vi "DDS_Clock.vi"() -> ()   [LabVIEW 2016] (continued)
"f1 [Hz] CH0"=312200000.0}, {"total time[ms]"=23.050000000000193, "f1 [Hz] CH0"=312200000.0}, {"total time[ms]"=23.100000000000193, "f1 [Hz] CH0"=312400000.0}, {"total time[ms]"=23.100000000000193, "f1 [Hz] CH0"=312400000.0}, {"total time[ms]"=23.150000000000194, "f1 [Hz] CH0"=312600000.0}, {"total time[ms]"=23.150000000000194, "f1 [Hz] CH0"=312600000.0}, {"total time[ms]"=23.200000000000195, "f1 [Hz] CH0"=312800000.0}, {"total time[ms]"=23.200000000000195, "f1 [Hz] CH0"=312800000.0}, {"total time[ms]"=23.250000000000195, "f1 [Hz] CH0"=313000000.0}, {"total time[ms]"=23.250000000000195, "f1 [Hz] CH0"=313000000.0}, {"total time[ms]"=23.300000000000196, "f1 [Hz] CH0"=313200000.0}, {"total time[ms]"=23.300000000000196, "f1 [Hz] CH0"=313200000.0}, {"total time[ms]"=23.350000000000197, "f1 [Hz] CH0"=313400000.0}, {"total time[ms]"=23.350000000000197, "f1 [Hz] CH0"=313400000.0}, {"total time[ms]"=23.400000000000198, "f1 [Hz] CH0"=313600000.0}, {"total time[ms]"=23.400000000000198, "f1 [Hz] CH0"=313600000.0}, {"total time[ms]"=23.4500000000002, "f1 [Hz] CH0"=313800000.0}, {"total time[ms]"=23.4500000000002, "f1 [Hz] CH0"=313800000.0}, {"total time[ms]"=23.5000000000002, "f1 [Hz] CH0"=314000000.0}, {"total time[ms]"=23.5000000000002, "f1 [Hz] CH0"=314000000.0}, {"total time[ms]"=23.5500000000002, "f1 [Hz] CH0"=314200000.0}, {"total time[ms]"=23.5500000000002, "f1 [Hz] CH0"=314200000.0}, {"total time[ms]"=23.6000000000002, "f1 [Hz] CH0"=314400000.0}, {"total time[ms]"=23.6000000000002, "f1 [Hz] CH0"=314400000.0}, {"total time[ms]"=23.6500000000002, "f1 [Hz] CH0"=314600000.0}, {"total time[ms]"=23.6500000000002, "f1 [Hz] CH0"=314600000.0}, {"total time[ms]"=23.700000000000202, "f1 [Hz] CH0"=314800000.0}, {"total time[ms]"=23.700000000000202, "f1 [Hz] CH0"=314800000.0}, {"total time[ms]"=23.750000000000203, "f1 [Hz] CH0"=315000000.0}, {"total time[ms]"=23.750000000000203, "f1 [Hz] CH0"=315000000.0}, {"total time[ms]"=23.800000000000203, "f1 [Hz] CH0"=315200000.0}, {"total time[ms]"=23.800000000000203, "f1 [Hz] CH0"=315200000.0}, {"total time[ms]"=23.850000000000204, "f1 [Hz] CH0"=315400000.0}, {"total time[ms]"=23.850000000000204, "f1 [Hz] CH0"=315400000.0}, {"total time[ms]"=23.900000000000205, "f1 [Hz] CH0"=315600000.0}, {"total time[ms]"=23.900000000000205, "f1 [Hz] CH0"=315600000.0}, {"total time[ms]"=23.950000000000205, "f1 [Hz] CH0"=315800000.0}, {"total time[ms]"=23.950000000000205, "f1 [Hz] CH0"=315800000.0}, {"total time[ms]"=24.000000000000206, "f1 [Hz] CH0"=316000000.0}, {"total time[ms]"=24.000000000000206, "f1 [Hz] CH0"=316000000.0}, {"total time[ms]"=24.050000000000207, "f1 [Hz] CH0"=316200000.0}, {"total time[ms]"=24.050000000000207, "f1 [Hz] CH0"=316200000.0}, {"total time[ms]"=24.100000000000207, "f1 [Hz] CH0"=316400000.0}, {"total time[ms]"=24.100000000000207, "f1 [Hz] CH0"=316400000.0}, {"total time[ms]"=24.150000000000208, "f1 [Hz] CH0"=316600000.0}, {"total time[ms]"=24.150000000000208, "f1 [Hz] CH0"=316600000.0}, {"total time[ms]"=24.20000000000021, "f1 [Hz] CH0"=316800000.0}, {"total time[ms]"=24.20000000000021, "f1 [Hz] CH0"=316800000.0}, {"total time[ms]"=24.25000000000021, "f1 [Hz] CH0"=317000000.0}, {"total time[ms]"=24.25000000000021, "f1 [Hz] CH0"=317000000.0}, {"total time[ms]"=24.30000000000021, "f1 [Hz] CH0"=317200000.0}, {"total time[ms]"=24.30000000000021, "f1 [Hz] CH0"=317200000.0}, {"total time[ms]"=24.35000000000021, "f1 [Hz] CH0"=317400000.0}, {"total time[ms]"=24.35000000000021, "f1 [Hz] CH0"=317400000.0}, {"total time[ms]"=24.40000000000021, "f1 [Hz] CH0"=317600000.0}, {"total time[ms]"=24.40000000000021, "f1 [Hz] CH0"=317600000.0}, {"total time[ms]"=24.450000000000212, "f1 [Hz] CH0"=317800000.0}, {"total time[ms]"=24.450000000000212, "f1 [Hz] CH0"=317800000.0}, {"total time[ms]"=24.500000000000213, "f1 [Hz] CH0"=318000000.0}, {"total time[ms]"=24.500000000000213, "f1 [Hz] CH0"=318000000.0}, {"total time[ms]"=24.550000000000214, "f1 [Hz] CH0"=318200000.0}, {"total time[ms]"=24.550000000000214, "f1 [Hz] CH0"=318200000.0}, {"total time[ms]"=24.600000000000215, "f1 [Hz] CH0"=318400000.0}, {"total time[ms]"=24.600000000000215, "f1 [Hz] CH0"=318400000.0}, {"total time[ms]"=24.650000000000215, "f1 [Hz] CH0"=318600000.0}, {"total time[ms]"=24.650000000000215, "f1 [Hz] CH0"=318600000.0}, {"total time[ms]"=24.700000000000216, "f1 [Hz] CH0"=318800000.0}, {"total time[ms]"=24.700000000000216, "f1 [Hz] CH0"=318800000.0}, {"total time[ms]"=24.750000000000217, "f1 [Hz] CH0"=319000000.0}, {"total time[ms]"=24.750000000000217, "f1 [Hz] CH0"=319000000.0}, {"total time[ms]"=24.800000000000217, "f1 [Hz] CH0"=319200000.0}, {"total time[ms]"=24.800000000000217, "f1 [Hz] CH0"=319200000.0}, {"total time[ms]"=24.850000000000218, "f1 [Hz] CH0"=319400000.0}, {"total time[ms]"=24.850000000000218, "f1 [Hz] CH0"=319400000.0}, {"total time[ms]"=24.90000000000022, "f1 [Hz] CH0"=319600000.0}, {"total time[ms]"=24.90000000000022, "f1 [Hz] CH0"=319600000.0}, {"total time[ms]"=24.95000000000022, "f1 [Hz] CH0"=319800000.0}, {"total time[ms]"=24.95000000000022, "f1 [Hz] CH0"=319800000.0}, {"total time[ms]"=25.00000000000022, "f1 [Hz] CH0"=320000000.0}, {"total time[ms]"=25.00000000000022, "f1 [Hz] CH0"=320000000.0}, {"total time[ms]"=25.05000000000022, "f1 [Hz] CH0"=319800000.0}, {"total time[ms]"=25.05000000000022, "f1 [Hz] CH0"=319800000.0}, {"total time[ms]"=25.10000000000022, "f1 [Hz] CH0"=319600000.0}, {"total time[ms]"=25.10000000000022, "f1 [Hz] CH0"=319600000.0}, {"total time[ms]"=25.150000000000222, "f1 [Hz] CH0"=319400000.0}, {"total time[ms]"=25.150000000000222, "f1 [Hz] CH0"=319400000.0}, {"total time[ms]"=25.200000000000223, "f1 [Hz] CH0"=319200000.0}, {"total time[ms]"=25.200000000000223, "f1 [Hz] CH0"=319200000.0}, {"total time[ms]"=25.250000000000224, "f1 [Hz] CH0"=319000000.0}, {"total time[ms]"=25.250000000000224, "f1 [Hz] CH0"=319000000.0}, {"total time[ms]"=25.300000000000225, "f1 [Hz] CH0"=318800000.0}, {"total time[ms]"=25.300000000000225, "f1 [Hz] CH0"=318800000.0}, {"total time[ms]"=25.350000000000225, "f1 [Hz] CH0"=318600000.0}, {"total time[ms]"=25.350000000000225, "f1 [Hz] CH0"=318600000.0}, {"total time[ms]"=25.400000000000226, "f1 [Hz] CH0"=318400000.0}, {"total time[ms]"=25.400000000000226, "f1 [Hz] CH0"=318400000.0}, {"total time[ms]"=25.450000000000227, "f1 [Hz] CH0"=318200000.0}, {"total time[ms]"=25.450000000000227, "f1 [Hz] CH0"=318200000.0}, {"total time[ms]"=25.500000000000227, "f1 [Hz] CH0"=318000000.0}, {"total time[ms]"=25.500000000000227, "f1 [Hz] CH0"=318000000.0}, {"total time[ms]"=25.550000000000228, "f1 [Hz] CH0"=317800000.0}, {"total time[ms]"=25.550000000000228, "f1 [Hz] CH0"=317800000.0}, {"total time[ms]"=25.60000000000023, "f1 [Hz] CH0"=317600000.0}, {"total time[ms]"=25.60000000000023, "f1 [Hz] CH0"=317600000.0}, {"total time[ms]"=25.65000000000023, "f1 [Hz] CH0"=317400000.0}, {"total time[ms]"=25.65000000000023, "f1 [Hz] CH0"=317400000.0}, {"total time[ms]"=25.70000000000023, "f1 [Hz] CH0"=317200000.0}, {"total time[ms]"=25.70000000000023, "f1 [Hz] CH0"=317200000.0}, {"total time[ms]"=25.75000000000023, "f1 [Hz] CH0"=317000000.0}, {"total time[ms]"=25.75000000000023, "f1 [Hz] CH0"=317000000.0}, {"total time[ms]"=25.80000000000023, "f1 [Hz] CH0"=316800000.0}, {"total time[ms]"=25.80000000000023, "f1 [Hz] CH0"=316800000.0}, {"total time[ms]"=25.850000000000232, "f1 [Hz] CH0"=316600000.0}, {"total time[ms]"=25.850000000000232, "f1 [Hz] CH0"=316600000.0}, {"total time[ms]"=25.900000000000233, "f1 [Hz] CH0"=316400000.0}, {"total time[ms]"=25.900000000000233, "f1 [Hz] CH0"=316400000.0}, {"total time[ms]"=25.950000000000234, "f1 [Hz] CH0"=316200000.0}, {"total time[ms]"=25.950000000000234, "f1 [Hz] CH0"=316200000.0}, {"total time[ms]"=26.000000000000234, "f1 [Hz] CH0"=316000000.0}, {"total time[ms]"=26.000000000000234, "f1 [Hz] CH0"=316000000.0}, {"total time[ms]"=26.050000000000235, "f1 [Hz] CH0"=315800000.0}, {"total time[ms]"=26.050000000000235, "f1 [Hz] CH0"=315800000.0}, {"total time[ms]"=26.100000000000236, "f1 [Hz] CH0"=315600000.0}, {"total time[ms]"=26.100000000000236, "f1 [Hz] CH0"=315600000.0}, {"total time[ms]"=26.150000000000237, "f1 [Hz] CH0"=315400000.0}, {"total time[ms]"=26.150000000000237, "f1 [Hz] CH0"=315400000.0}, {"total time[ms]"=26.200000000000237, "f1 [Hz] CH0"=315200000.0}, {"total time[ms]"=26.200000000000237, "f1 [Hz] CH0"=315200000.0}, {"total time[ms]"=26.250000000000238, "f1 [Hz] CH0"=315000000.0}, {"total time[ms]"=26.250000000000238, "f1 [Hz] CH0"=315000000.0}, {"total time[ms]"=26.30000000000024, "f1 [Hz] CH0"=314800000.0}, {"total time[ms]"=26.30000000000024, "f1 [Hz] CH0"=314800000.0}, {"total time[ms]"=26.35000000000024, "f1 [Hz] CH0"=314600000.0}, {"total time[ms]"=26.35000000000024, "f1 [Hz] CH0"=314600000.0}, {"total time[ms]"=26.40000000000024, "f1 [Hz] CH0"=314400000.0}, {"total time[ms]"=26.40000000000024, "f1 [Hz] CH0"=314400000.0}, {"total time[ms]"=26.45000000000024, "f1 [Hz] CH0"=314200000.0}, {"total time[ms]"=26.45000000000024, "f1 [Hz] CH0"=314200000.0}, {"total time[ms]"=26.50000000000024, "f1 [Hz] CH0"=314000000.0}, {"total time[ms]"=26.50000000000024, "f1 [Hz] CH0"=314000000.0}, {"total time[ms]"=26.550000000000242, "f1 [Hz] CH0"=313800000.0}, {"total time[ms]"=26.550000000000242, "f1 [Hz] CH0"=313800000.0}, {"total time[ms]"=26.600000000000243, "f1 [Hz] CH0"=313600000.0}, {"total time[ms]"=26.600000000000243, "f1 [Hz] CH0"=313600000.0}, {"total time[ms]"=26.650000000000244, "f1 [Hz] CH0"=313400000.0}, {"total time[ms]"=26.650000000000244, "f1 [Hz] CH0"=313400000.0}, {"total time[ms]"=26.700000000000244, "f1 [Hz] CH0"=313200000.0}, {"total time[ms]"=26.700000000000244, "f1 [Hz] CH0"=313200000.0}, {"total time[ms]"=26.750000000000245, "f1 [Hz] CH0"=313000000.0}, {"total time[ms]"=26.750000000000245, "f1 [Hz] CH0"=313000000.0}, {"total time[ms]"=26.800000000000246, "f1 [Hz] CH0"=312800000.0}, {"total time[ms]"=26.800000000000246, "f1 [Hz] CH0"=312800000.0}, {"total time[ms]"=26.850000000000247, "f1 [Hz] CH0"=312600000.0}, {"total time[ms]"=26.850000000000247, "f1 [Hz] CH0"=312600000.0}, {"total time[ms]"=26.900000000000247, "f1 [Hz] CH0"=312400000.0}, {"total time[ms]"=26.900000000000247, "f1 [Hz] CH0"=312400000.0}, {"total time[ms]"=26.950000000000248, "f1 [Hz] CH0"=312200000.0}, {"total time[ms]"=26.950000000000248, "f1 [Hz] CH0"=312200000.0}, {"total time[ms]"=27.00000000000025, "f1 [Hz] CH0"=312000000.0}, {"total time[ms]"=27.00000000000025, "f1 [Hz] CH0"=312000000.0}, {"total time[ms]"=27.05000000000025, "f1 [Hz] CH0"=311800000.0}, {"total time[ms]"=27.05000000000025, "f1 [Hz] CH0"=311800000.0}, {"total time[ms]"=27.10000000000025, "f1 [Hz] CH0"=311600000.0}, {"total time[ms]"=27.10000000000025, "f1 [Hz] CH0"=311600000.0}, {"total time[ms]"=27.15000000000025, "f1 [Hz] CH0"=311400000.0}, {"total time[ms]"=27.15000000000025, "f1 [Hz] CH0"=311400000.0}, {"total time[ms]"=27.20000000000025, "f1 [Hz] CH0"=311200000.0}, {"total time[ms]"=27.20000000000025, "f1 [Hz] CH0"=311200000.0}, {"total time[ms]"=27.250000000000252, "f1 [Hz] CH0"=311000000.0}, {"total time[ms]"=27.250000000000252, "f1 [Hz] CH0"=311000000.0}, {"total time[ms]"=27.300000000000253, "f1 [Hz] CH0"=310800000.0}, {"total time[ms]"=27.300000000000253, "f1 [Hz] CH0"=310800000.0}, {"total time[ms]"=27.350000000000254, "f1 [Hz] CH0"=310600000.0}, {"total time[ms]"=27.350000000000254, "f1 [Hz] CH0"=310600000.0}, {"total time[ms]"=27.400000000000254, "f1 [Hz] CH0"=310400000.0}, {"total time[ms]"=27.400000000000254, "f1 [Hz] CH0"=310400000.0}, {"total time[ms]"=27.450000000000255, "f1 [Hz] CH0"=310200000.0}, {"total time[ms]"=27.450000000000255, "f1 [Hz] CH0"=310200000.0}, {"total time[ms]"=27.500000000000256, "f1 [Hz] CH0"=310000000.0}, {"total time[ms]"=27.500000000000256, "f1 [Hz] CH0"=310000000.0}, {"total time[ms]"=27.550000000000257, "f1 [Hz] CH0"=309800000.0}, {"total time[ms]"=27.550000000000257, "f1 [Hz] CH0"=309800000.0}, {"total time[ms]"=27.600000000000257, "f1 [Hz] CH0"=309600000.0}, {"total time[ms]"=27.600000000000257, "f1 [Hz] CH0"=309600000.0}, {"total time[ms]"=27.650000000000258, "f1 [Hz] CH0"=309400000.0}, {"total time[ms]"=27.650000000000258, "f1 [Hz] CH0"=309400000.0}, {"total time[ms]"=27.70000000000026, "f1 [Hz] CH0"=309200000.0}, {"total time[ms]"=27.70000000000026, "f1 [Hz] CH0"=309200000.0}, {"total time[ms]"=27.75000000000026, "f1 [Hz] CH0"=309000000.0}, {"total time[ms]"=27.75000000000026, "f1 [Hz] CH0"=309000000.0}, {"total time[ms]"=27.80000000000026, "f1 [Hz] CH0"=308800000.0}, {"total time[ms]"=27.80000000000026, "f1 [Hz] CH0"=308800000.0}, {"total time[ms]"=27.85000000000026, "f1 [Hz] CH0"=308600000.0}, {"total time[ms]"=27.85000000000026, "f1 [Hz] CH0"=308600000.0}, {"total time[ms]"=27.90000000000026, "f1 [Hz] CH0"=308400000.0}, {"total time[ms]"=27.90000000000026, "f1 [Hz] CH0"=308400000.0}, {"total time[ms]"=27.950000000000262, "f1 [Hz] CH0"=308200000.0}, {"total time[ms]"=27.950000000000262, "f1 [Hz] CH0"=308200000.0}, {"total time[ms]"=28.000000000000263, "f1 [Hz] CH0"=308000000.0}, {"total time[ms]"=28.000000000000263, "f1 [Hz] CH0"=308000000.0}, {"total time[ms]"=28.050000000000264, "f1 [Hz] CH0"=307800000.0}, {"total time[ms]"=28.050000000000264, "f1 [Hz] CH0"=307800000.0}, {"total time[ms]"=28.100000000000264, "f1 [Hz] CH0"=307600000.0}, {"total time[ms]"=28.100000000000264, "f1 [Hz] CH0"=307600000.0}, {"total time[ms]"=28.150000000000265, "f1 [Hz] CH0"=307400000.0}, {"total time[ms]"=28.150000000000265, "f1 [Hz] CH0"=307400000.0}, {"total time[ms]"=28.200000000000266, "f1 [Hz] CH0"=307200000.0}, {"total time[ms]"=28.200000000000266, "f1 [Hz] CH0"=307200000.0}, {"total time[ms]"=28.250000000000266, "f1 [Hz] CH0"=307000000.0}, {"total time[ms]"=28.250000000000266, "f1 [Hz] CH0"=307000000.0}, {"total time[ms]"=28.300000000000267, "f1 [Hz] CH0"=306800000.0}, {"total time[ms]"=28.300000000000267, "f1 [Hz] CH0"=306800000.0}, {"total time[ms]"=28.350000000000268, "f1 [Hz] CH0"=306600000.0}, {"total time[ms]"=28.350000000000268, "f1 [Hz] CH0"=306600000.0}, {"total time[ms]"=28.40000000000027, "f1 [Hz] CH0"=306400000.0}, {"total time[ms]"=28.40000000000027, "f1 [Hz] CH0"=306400000.0}, {"total time[ms]"=28.45000000000027, "f1 [Hz] CH0"=306200000.0}, {"total time[ms]"=28.45000000000027, "f1 [Hz] CH0"=306200000.0}, {"total time[ms]"=28.50000000000027, "f1 [Hz] CH0"=306000000.0}, {"total time[ms]"=28.50000000000027, "f1 [Hz] CH0"=306000000.0}, {"total time[ms]"=28.55000000000027, "f1 [Hz] CH0"=305800000.0}, {"total time[ms]"=28.55000000000027, "f1 [Hz] CH0"=305800000.0}, {"total time[ms]"=28.60000000000027, "f1 [Hz] CH0"=305600000.0}, {"total time[ms]"=28.60000000000027, "f1 [Hz] CH0"=305600000.0}, {"total time[ms]"=28.650000000000272, "f1 [Hz] CH0"=305400000.0}, {"total time[ms]"=28.650000000000272, "f1 [Hz] CH0"=305400000.0}, {"total time[ms]"=28.700000000000273, "f1 [Hz] CH0"=305200000.0}, {"total time[ms]"=28.700000000000273, "f1 [Hz] CH0"=305200000.0}, {"total time[ms]"=28.750000000000274, "f1 [Hz] CH0"=305000000.0}, {"total time[ms]"=28.750000000000274, "f1 [Hz] CH0"=305000000.0}, {"total time[ms]"=28.800000000000274, "f1 [Hz] CH0"=304800000.0}, {"total time[ms]"=28.800000000000274, "f1 [Hz] CH0"=304800000.0}, {"total time[ms]"=28.850000000000275, "f1 [Hz] CH0"=304600000.0}, {"total time[ms]"=28.850000000000275, "f1 [Hz] CH0"=304600000.0}, {"total time[ms]"=28.900000000000276, "f1 [Hz] CH0"=304400000.0}, {"total time[ms]"=28.900000000000276, "f1 [Hz] CH0"=304400000.0}, {"total time[ms]"=28.950000000000276, "f1 [Hz] CH0"=304200000.0}, {"total time[ms]"=28.950000000000276, "f1 [Hz] CH0"=304200000.0}, {"total time[ms]"=29.000000000000277, "f1 [Hz] CH0"=304000000.0}, {"total time[ms]"=29.000000000000277, "f1 [Hz] CH0"=304000000.0}, {"total time[ms]"=29.050000000000278, "f1 [Hz] CH0"=303800000.0}, {"total time[ms]"=29.050000000000278, "f1 [Hz] CH0"=303800000.0}, {"total time[ms]"=29.10000000000028, "f1 [Hz] CH0"=303600000.0}, {"total time[ms]"=29.10000000000028, "f1 [Hz] CH0"=303600000.0}, {"total time[ms]"=29.15000000000028, "f1 [Hz] CH0"=303400000.0}, {"total time[ms]"=29.15000000000028, "f1 [Hz] CH0"=303400000.0}, {"total time[ms]"=29.20000000000028, "f1 [Hz] CH0"=303200000.0}, {"total time[ms]"=29.20000000000028, "f1 [Hz] CH0"=303200000.0}, {"total time[ms]"=29.25000000000028, "f1 [Hz] CH0"=303000000.0}, {"total time[ms]"=29.25000000000028, "f1 [Hz] CH0"=303000000.0}, {"total time[ms]"=29.30000000000028, "f1 [Hz] CH0"=302800000.0}, {"total time[ms]"=29.30000000000028, "f1 [Hz] CH0"=302800000.0}, {"total time[ms]"=29.350000000000282, "f1 [Hz] CH0"=302600000.0}, {"total time[ms]"=29.350000000000282, "f1 [Hz] CH0"=302600000.0}, {"total time[ms]"=29.400000000000283, "f1 [Hz] CH0"=302400000.0}, {"total time[ms]"=29.400000000000283, "f1 [Hz] CH0"=302400000.0}, {"total time[ms]"=29.450000000000284, "f1 [Hz] CH0"=302200000.0}, {"total time[ms]"=29.450000000000284, "f1 [Hz] CH0"=302200000.0}, {"total time[ms]"=29.500000000000284, "f1 [Hz] CH0"=302000000.0}, {"total time[ms]"=29.500000000000284, "f1 [Hz] CH0"=302000000.0}, {"total time[ms]"=29.550000000000285, "f1 [Hz] CH0"=301800000.0}, {"total time[ms]"=29.550000000000285, "f1 [Hz] CH0"=301800000.0}, {"total time[ms]"=29.600000000000286, "f1 [Hz] CH0"=301600000.0}, {"total time[ms]"=29.600000000000286, "f1 [Hz] CH0"=301600000.0}, {"total time[ms]"=29.650000000000286, "f1 [Hz] CH0"=301400000.0}, {"total time[ms]"=29.650000000000286, "f1 [Hz] CH0"=301400000.0}, {"total time[ms]"=29.700000000000287, "f1 [Hz] CH0"=301200000.0}, {"total time[ms]"=29.700000000000287, "f1 [Hz] CH0"=301200000.0}, {"total time[ms]"=29.750000000000288, "f1 [Hz] CH0"=301000000.0}, {"total time[ms]"=29.750000000000288, "f1 [Hz] CH0"=301000000.0}, {"total time[ms]"=29.80000000000029, "f1 [Hz] CH0"=300800000.0}, {"total time[ms]"=29.80000000000029, "f1 [Hz] CH0"=300800000.0}, {"total time[ms]"=29.85000000000029, "f1 [Hz] CH0"=300600000.0}, {"total time[ms]"=29.85000000000029, "f1 [Hz] CH0"=300600000.0}, {"total time[ms]"=29.90000000000029, "f1 [Hz] CH0"=300400000.0}, {"total time[ms]"=29.90000000000029, "f1 [Hz] CH0"=300400000.0}, {"total time[ms]"=29.95000000000029, "f1 [Hz] CH0"=300200000.0}, {"total time[ms]"=29.95000000000029, "f1 [Hz] CH0"=300200000.0}, {"total time[ms]"=30.00000000000029, "f1 [Hz] CH0"=300000000.0}, {"total time[ms]"=30.00000000000029, "f1 [Hz] CH0"=300000000.0}, {"total time[ms]"=30.050000000000292, "f1 [Hz] CH0"=300200000.0}, {"total time[ms]"=30.050000000000292, "f1 [Hz] CH0"=300200000.0}, {"total time[ms]"=30.100000000000293, "f1 [Hz] CH0"=300400000.0}, {"total time[ms]"=30.100000000000293, "f1 [Hz] CH0"=300400000.0}, {"total time[ms]"=30.150000000000293, "f1 [Hz] CH0"=300600000.0}, {"total time[ms]"=30.150000000000293, "f1 [Hz] CH0"=300600000.0}, {"total time[ms]"=30.200000000000294, "f1 [Hz] CH0"=300800000.0}, {"total time[ms]"=30.200000000000294, "f1 [Hz] CH0"=300800000.0}, {"total time[ms]"=30.250000000000295, "f1 [Hz] CH0"=301000000.0}, {"total time[ms]"=30.250000000000295, "f1 [Hz] CH0"=301000000.0}, {"total time[ms]"=30.300000000000296, "f1 [Hz] CH0"=301200000.0}, {"total time[ms]"=30.300000000000296, "f1 [Hz] CH0"=301200000.0}, {"total time[ms]"=30.350000000000296, "f1 [Hz] CH0"=301400000.0}, {"total time[ms]"=30.350000000000296, "f1 [Hz] CH0"=301400000.0}, {"total time[ms]"=30.400000000000297, "f1 [Hz] CH0"=301600000.0}, {"total time[ms]"=30.400000000000297, "f1 [Hz] CH0"=301600000.0}, {"total time[ms]"=30.450000000000298, "f1 [Hz] CH0"=301800000.0}, {"total time[ms]"=30.450000000000298, "f1 [Hz] CH0"=301800000.0}, {"total time[ms]"=30.5000000000003, "f1 [Hz] CH0"=302000000.0}, {"total time[ms]"=30.5000000000003, "f1 [Hz] CH0"=302000000.0}, {"total time[ms]"=30.5500000000003, "f1 [Hz] CH0"=302200000.0}, {"total time[ms]"=30.5500000000003, "f1 [Hz] CH0"=302200000.0}, {"total time[ms]"=30.6000000000003, "f1 [Hz] CH0"=302400000.0}, {"total time[ms]"=30.6000000000003, "f1 [Hz] CH0"=302400000.0}, {"total time[ms]"=30.6500000000003, "f1 [Hz] CH0"=302600000.0}, {"total time[ms]"=30.6500000000003, 
